vi "Get Channels Array.vi"(0 "TDMS File Reference in":refnum<k34>, 11 "error in (no error)":errorcluster, 12 "Filtering Settings":T1={"Filtered Groups"=[], "Group Filter Mode"=enum."Exclude", "Group Filter Regex?"=FALSE, "Filtered Channels"=[], "Channel Filter Mode"=enum."Exclude", "Channel Filter Regex?"=FALSE, "Filter Time Start"=timestamp(0 s since 1904-01-01), "Filter Time End"=timestamp(0 s since 1904-01-01), "Time Filter Mode"=enum."Include", "Time Filter Enabled"=FALSE}) -> (4 "TDMS File Reference out":refnum<k34>, 10 "Group/Channel Names":string[](array[string]), 15 "error out":errorcluster)   [LabVIEW 2017, in "XTree.xctl"]
doc: "Creates a list of groups and channels, according to the specified filter settings."
uses:
  <vilib>/addons/_NIFileIO/XTree/XTree.xctl
  <vilib>/addons/_NIFileIO/XTree/Controls/Filter Settings.ctl
  <vilib>/addons/_NIFileIO/XTree/Controls/Filter Mode.ctl
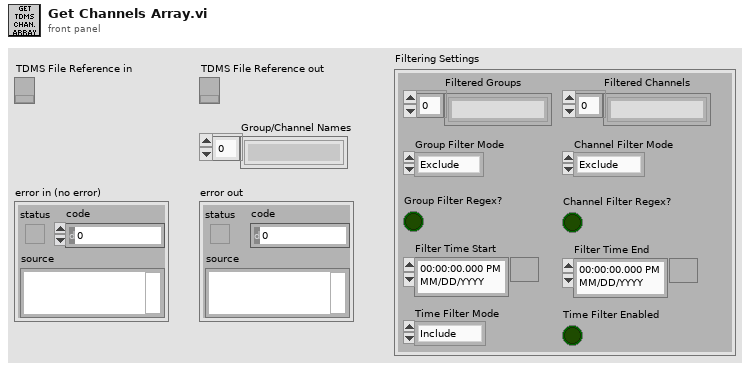
[diagram p1: front panel]
types:
  T1 = typedef "XTree.xctl/Filter Settings.ctl" = cluster{"Filtered Groups":string[], "Group Filter Mode":T2, "Group Filter Regex?":bool, "Filtered Channels":string[], "Channel Filter Mode":T2, "Channel Filter Regex?":bool, "Filter Time Start":timestamp, "Filter Time End":timestamp, "Time Filter Mode":T2, "Time Filter Enabled":bool}
  T2 = typedef "XTree.xctl/Filter Mode.ctl" = enum16{"Exclude", "Include"}
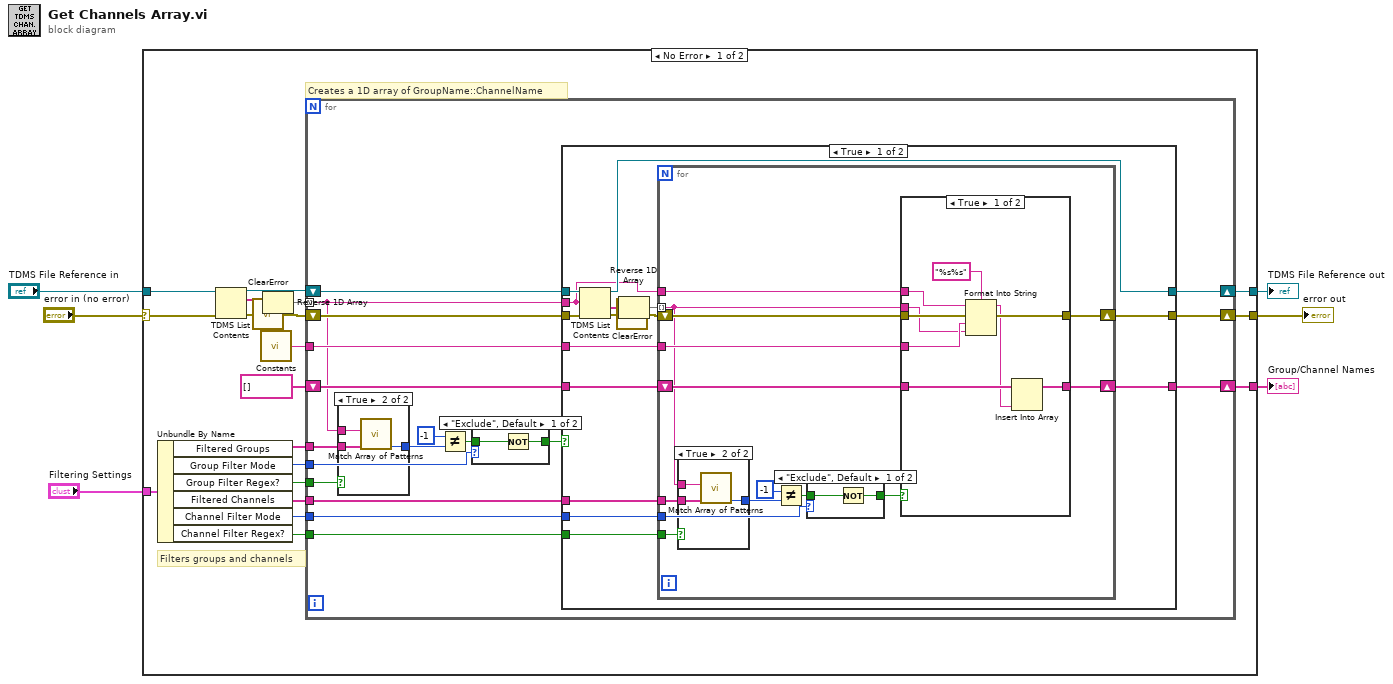
[diagram p0: block diagram]
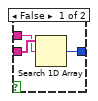
[diagram p2: hidden frame]
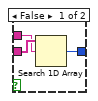
[diagram p4: hidden frame]
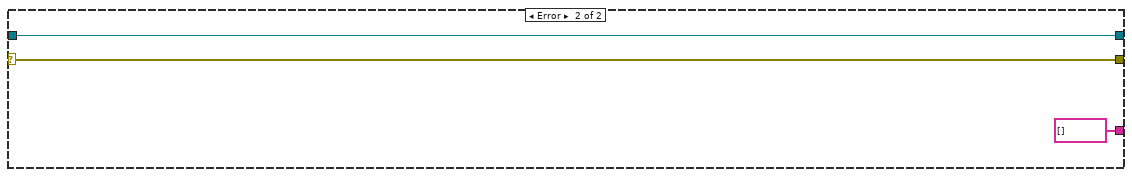
[diagram p8: hidden frame]
diagram:
  n1 = case shown="No Error" "error in (no error)" {
    selector: "error in (no error)" -> [w8 w106]
    tunnel: "TDMS File Reference in" -> [w24 w107]
    tunnel: [w22 w107] -> w5
    tunnel: [w21 w106] -> w4
    tunnel: [w16 string[] []] -> w3
    tunnel: "Filtering Settings" -> [w15 _]
    frame No Error {
      # "Filters groups and channels"
      # "Creates a 1D array of GroupName::ChannelName"
      n2 = Unbundle By Name(w15) -> ("Filtered Groups"=w14:string[], "Group Filter Mode"=w13:T2, "Group Filter Regex?"=w10:bool, "Filtered Channels"=w11:string[], "Channel Filter Mode"=w12:T2, "Channel Filter Regex?"=w9:bool)
      n3 = TDMS List Contents(4:w8, 7:w24) -> (0:w7:errorcluster, 2:w20:string[], 3:w18:refnum<k34>)  [unwired: 1 in, 1 out]
      n4 = call <vilib>:"ClearError.vi"("error in (no error)"=w7) -> ("error out"=w23:errorcluster)
      n5 = call <vilib>:"Constants.vi"() -> ("String Delimeter"=w25:string)  [unwired: 5 in]
      n6 = Reverse 1D Array(array=w20) -> (reversed array=w19:string[])
      n7 = for {
        tunnel: w19 -> [w33] mode=indexing
        shift-right: [w37] -> w21
        shift-left: w23 -> [w43]
        shift-right: [w42] -> w22
        shift-left: w18 -> [w41]
        shift-right: [w39] -> w16
        shift-left: string[] [] -> [w40]
        tunnel: w25 -> [w38]
        tunnel: w13 -> [w32]
        tunnel: w14 -> [w34]
        tunnel: w12 -> [w36]
        tunnel: w11 -> [w35]
        tunnel: w10 -> [w27]
        tunnel: w9 -> [w26]
        n8 = case shown="True" w27 {
          tunnel: w34 -> [w46 w49]
          tunnel: w33 -> [w45 w48]
          tunnel: [w44 w47] -> w30
          frame False {
            n9 = Search 1D Array(1D array=w46, element=w45) -> (index of element=w44:i32)  [unwired: 1 in]
          }
          frame True {
            n10 = call <vilib>:"Match Array of Patterns.vi"("Patterns"=w49, "String"=w48) -> ("Index of element"=w47:i32)  [unwired: 8 in, 1 out]
          }
        }
        n11 = Not Equal?(x=-1, y=w30) -> (x != y?=w28:bool)
        n12 = case shown="\"Exclude\", Default" w32 {
          tunnel: w28 -> [w50 w52]
          tunnel: [w51 w52] -> w31
          frame "Exclude", Default {
            n13 = Not(x=w50) -> (.not. x?=w51:bool)
          }
          frame "Include" {
          }
        }
        n14 = case shown="True" w31 {
          tunnel: w43 -> [w67 w103]
          tunnel: [w66 w104] -> w42
          tunnel: w41 -> [w65 w104]
          tunnel: w40 -> [w56 w102]
          tunnel: [w55 w102] -> w39
          tunnel: w38 -> [w62 _]
          tunnel: [w60 w103] -> w37
          tunnel: w33 -> [w59 _]
          tunnel: w36 -> [w58 _]
          tunnel: w35 -> [w57 _]
          tunnel: w26 -> [w54 _]
          frame True {
            n15 = TDMS List Contents(4:w67, 6:w59, 7:w65) -> (0:w53:errorcluster, 1:w63:string[], 3:w66:refnum<k34>)  [unwired: 1 out]
            n16 = call <vilib>:"ClearError.vi"("error in (no error)"=w53) -> ("error out"=w61:errorcluster)
            n17 = Reverse 1D Array(array=w63) -> (reversed array=w64:string[])
            n18 = for {
              tunnel: w64 -> [w73] mode=indexing
              tunnel: w59 -> [w81]
              tunnel: w62 -> [w80]
              shift-right: [w78] -> w60
              shift-left: w61 -> [w79]
              tunnel: w58 -> [w74]
              tunnel: w57 -> [w72]
              shift-right: [w76] -> w55
              shift-left: w56 -> [w77]
              tunnel: w54 -> [w68]
              n19 = case shown="True" w68 {
                tunnel: w72 -> [w84 w87]
                tunnel: w73 -> [w83 w86]
                tunnel: [w82 w85] -> w70
                frame False {
                  n20 = Search 1D Array(1D array=w84, element=w83) -> (index of element=w82:i32)  [unwired: 1 in]
                }
                frame True {
                  n21 = call <vilib>:"Match Array of Patterns.vi"("Patterns"=w87, "String"=w86) -> ("Index of element"=w85:i32)  [unwired: 8 in, 1 out]
                }
              }
              n22 = Not Equal?(x=-1, y=w70) -> (x != y?=w69:bool)
              n23 = case shown="\"Exclude\", Default" w74 {
                tunnel: w69 -> [w88 w90]
                tunnel: [w89 w90] -> w75
                frame "Exclude", Default {
                  n24 = Not(x=w88) -> (.not. x?=w89:bool)
                }
                frame "Include" {
                }
              }
              n25 = case shown="True" w75 {
                tunnel: w81 -> [w99 _]
                tunnel: w80 -> [w98 _]
                tunnel: w79 -> [w96 w101]
                tunnel: [w95 w101] -> w78
                tunnel: w73 -> [w94 _]
                tunnel: w77 -> [w93 w100]
                tunnel: [w91 w100] -> w76
                frame True {
                  n26 = Format Into String(format string="%s%s", initial string=w99, error in=w96, w98, w94) -> (resulting string=w92:string, error out=w95:errorcluster)
                  n27 = Insert Into Array(array=w93, new element=w92) -> (w91:string[])  [unwired: 1 in]
                }
                frame False {
                }
              }
            }
          }
          frame False {
          }
        }
      }
    }
    frame Error {
    }
  }
  "TDMS File Reference out" <- w5
  "error out" <- w4
  "Group/Channel Names" <- w3
